vi "PV_DataLog.vi"(0 "Start 2":bool=TRUE, 2 "Start":bool=TRUE) -> ()   [LabVIEW 2016]
uses:
  <vilib>/Utility/file.llb/Write Delimited Spreadsheet (DBL).vi
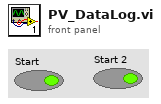
[diagram p1: front panel]
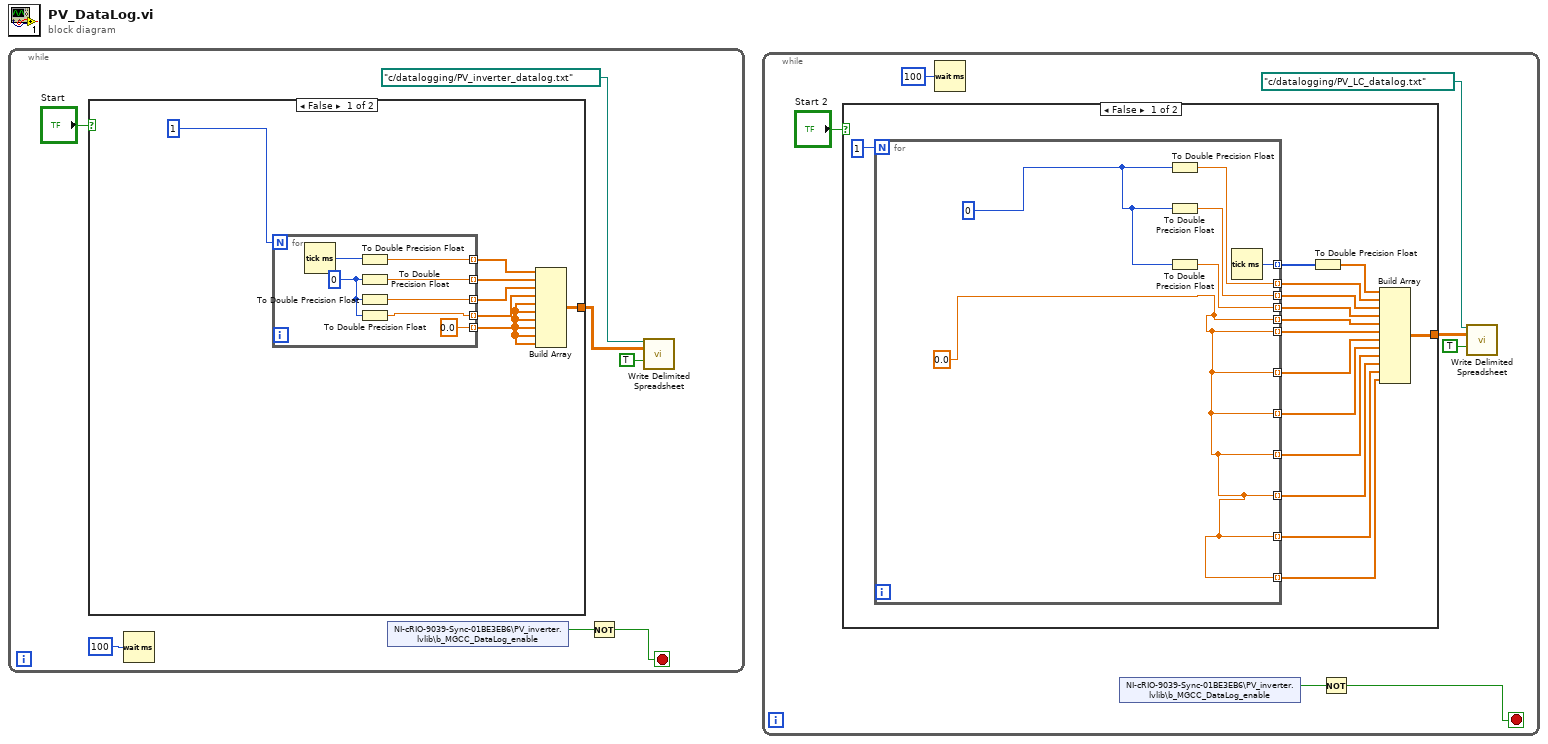
[diagram p0: block diagram]
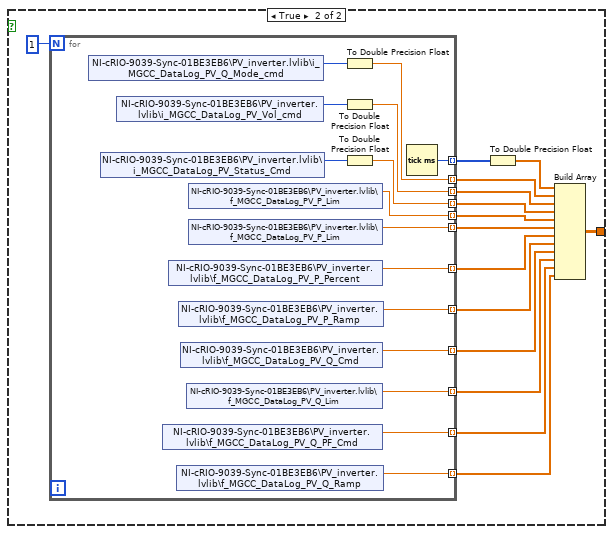
[diagram p2: hidden frame]
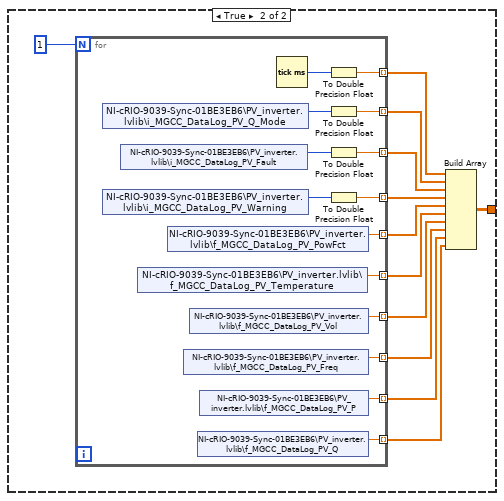
[diagram p3: hidden frame]
diagram:
  n1 = while {
    stop <- w1 stop-if-true
    n2 = case shown="False" "Start" {
      tunnel: [w9 w23] -> w4
      frame False {
        n3 = for {
          N: 1 -> [_]
          tunnel: [w21] -> w14 mode=indexing
          tunnel: [w19] -> w13 mode=indexing
          tunnel: [w18] -> w12 mode=indexing
          tunnel: [0.0] -> w11 mode=indexing
          tunnel: [w16] -> w10 mode=indexing
          w20 = 0
          n4 = Tick Count (ms)() -> (millisecond timer value=w15:u32)
          n5 = To Double Precision Float(number=w15) -> (double precision float=w16:dbl)
          n6 = To Double Precision Float(number=w20) -> (double precision float=w21:dbl)
          n7 = To Double Precision Float(number=w20) -> (double precision float=w19:dbl)
          n8 = To Double Precision Float(number=w20) -> (double precision float=w18:dbl)
        }
        n9 = Build Array(w10, w14, w13, w12, w11, w11, w11, w11, w11, w11) -> (w9:dbl[][])
      }
      frame True {
        n10 = for {
          N: 1 -> [_]
          tunnel: [w47] -> w33 mode=indexing
          tunnel: [w46] -> w32 mode=indexing
          tunnel: [w45] -> w31 mode=indexing
          tunnel: [w44] -> w30 mode=indexing
          tunnel: [w43] -> w29 mode=indexing
          tunnel: [w42] -> w28 mode=indexing
          tunnel: [w39] -> w27 mode=indexing
          tunnel: [w37] -> w26 mode=indexing
          tunnel: [w36] -> w25 mode=indexing
          tunnel: [w35] -> w24 mode=indexing
          n11 = shared-variable "NI-cRIO-9039-Sync-01BE3EB6\\PV_inverter.lvlib\\i_MGCC_DataLog_PV_Q_Mode"() -> (w41:i16)  [unwired: 1 in, 1 out]
          n12 = shared-variable "NI-cRIO-9039-Sync-01BE3EB6\\PV_inverter.lvlib\\i_MGCC_DataLog_PV_Warning"() -> (w38:i16)  [unwired: 1 in, 1 out]
          n13 = shared-variable "NI-cRIO-9039-Sync-01BE3EB6\\PV_inverter.lvlib\\i_MGCC_DataLog_PV_Fault"() -> (w40:i16)  [unwired: 1 in, 1 out]
          n14 = shared-variable "NI-cRIO-9039-Sync-01BE3EB6\\PV_inverter.lvlib\\f_MGCC_DataLog_PV_Temperature"() -> (w47:dbl)  [unwired: 1 in, 1 out]
          n15 = shared-variable "NI-cRIO-9039-Sync-01BE3EB6\\PV_inverter.lvlib\\f_MGCC_DataLog_PV_PowFct"() -> (w36:dbl)  [unwired: 1 in, 1 out]
          n16 = shared-variable "NI-cRIO-9039-Sync-01BE3EB6\\PV_inverter.lvlib\\f_MGCC_DataLog_PV_Freq"() -> (w45:dbl)  [unwired: 1 in, 1 out]
          n17 = shared-variable "NI-cRIO-9039-Sync-01BE3EB6\\PV_inverter.lvlib\\f_MGCC_DataLog_PV_Vol"() -> (w46:dbl)  [unwired: 1 in, 1 out]
          n18 = shared-variable "NI-cRIO-9039-Sync-01BE3EB6\\PV_inverter.lvlib\\f_MGCC_DataLog_PV_Q"() -> (w43:dbl)  [unwired: 1 in, 1 out]
          n19 = shared-variable "NI-cRIO-9039-Sync-01BE3EB6\\PV_inverter.lvlib\\f_MGCC_DataLog_PV_P"() -> (w44:dbl)  [unwired: 1 in, 1 out]
          n20 = Tick Count (ms)() -> (millisecond timer value=w34:u32)
          n21 = To Double Precision Float(number=w34) -> (double precision float=w35:dbl)
          n22 = To Double Precision Float(number=w41) -> (double precision float=w42:dbl)
          n23 = To Double Precision Float(number=w40) -> (double precision float=w39:dbl)
          n24 = To Double Precision Float(number=w38) -> (double precision float=w37:dbl)
        }
        n25 = Build Array(w24, w28, w27, w26, w25, w33, w32, w31, w30, w29) -> (w23:dbl[][])
      }
    }
    n26 = Wait (ms)(milliseconds to wait=u32 100) -> ()  [unwired: 1 out]
    n27 = shared-variable "NI-cRIO-9039-Sync-01BE3EB6\\PV_inverter.lvlib\\b_MGCC_DataLog_enable"() -> (w2:bool)  [unwired: 1 in, 1 out]
    n28 = Not(x=w2) -> (.not. x?=w1:bool)
    n29 = call-poly <vilib>:"Write Delimited Spreadsheet.vi"("file path (dialog if empty)"=path "c:/datalogging/PV_inverter_datalog.txt", "2D data"=w4, "append to file? (new file:F)"=TRUE) -> ()  [unwired: 11 in, 2 out]
  }
  n30 = while {
    stop <- w48 stop-if-true
    n31 = case shown="False" "Start 2" {
      tunnel: [w55 w83] -> w53
      frame False {
        n32 = for {
          N: 1 -> [_]
          tunnel: [w75] -> w57 mode=indexing
          tunnel: [w73] -> w59 mode=indexing
          tunnel: [w70] -> w68 mode=indexing
          tunnel: [w70] -> w67 mode=indexing
          tunnel: [w70] -> w66 mode=indexing
          tunnel: [w70] -> w65 mode=indexing
          tunnel: [w70] -> w64 mode=indexing
          tunnel: [w74] -> w63 mode=indexing
          tunnel: [w70] -> w62 mode=indexing
          tunnel: [w70] -> w61 mode=indexing
          tunnel: [w70] -> w60 mode=indexing
          tunnel: [w72] -> w58 mode=indexing
          w70 = 0.0
          w71 = 0
          n33 = To Double Precision Float(number=w71) -> (double precision float=w74:dbl)
          n34 = To Double Precision Float(number=w71) -> (double precision float=w73:dbl)
          n35 = To Double Precision Float(number=w71) -> (double precision float=w72:dbl)
          n36 = Tick Count (ms)() -> (millisecond timer value=w75:u32)
        }
        n37 = To Double Precision Float(number=w57) -> (double precision float=w56:dbl[])
        n38 = Build Array(w56, w63, w59, w58, w68, w67, w66, w65, w64, w62, w61, w60) -> (w55:dbl[][])
      }
      frame True {
        n39 = for {
          N: 1 -> [_]
          tunnel: [w105] -> w77 mode=indexing
          tunnel: [w92] -> w79 mode=indexing
          tunnel: [w104] -> w89 mode=indexing
          tunnel: [w103] -> w88 mode=indexing
          tunnel: [w102] -> w87 mode=indexing
          tunnel: [w101] -> w86 mode=indexing
          tunnel: [w100] -> w85 mode=indexing
          tunnel: [w93] -> w84 mode=indexing
          tunnel: [w99] -> w82 mode=indexing
          tunnel: [w98] -> w81 mode=indexing
          tunnel: [w97] -> w80 mode=indexing
          tunnel: [w91] -> w78 mode=indexing
          n40 = shared-variable "NI-cRIO-9039-Sync-01BE3EB6\\PV_inverter.lvlib\\i_MGCC_DataLog_PV_Q_Mode_cmd"() -> (w96:i16)  [unwired: 1 in, 1 out]
          n41 = shared-variable "NI-cRIO-9039-Sync-01BE3EB6\\PV_inverter.lvlib\\i_MGCC_DataLog_PV_Status_Cmd"() -> (w95:i16)  [unwired: 1 in, 1 out]
          n42 = shared-variable "NI-cRIO-9039-Sync-01BE3EB6\\PV_inverter.lvlib\\i_MGCC_DataLog_PV_Vol_cmd"() -> (w94:i16)  [unwired: 1 in, 1 out]
          n43 = shared-variable "NI-cRIO-9039-Sync-01BE3EB6\\PV_inverter.lvlib\\f_MGCC_DataLog_PV_Q_PF_Cmd"() -> (w98:dbl)  [unwired: 1 in, 1 out]
          n44 = shared-variable "NI-cRIO-9039-Sync-01BE3EB6\\PV_inverter.lvlib\\f_MGCC_DataLog_PV_P_Percent"() -> (w102:dbl)  [unwired: 1 in, 1 out]
          n45 = shared-variable "NI-cRIO-9039-Sync-01BE3EB6\\PV_inverter.lvlib\\f_MGCC_DataLog_PV_Q_Ramp"() -> (w97:dbl)  [unwired: 1 in, 1 out]
          n46 = shared-variable "NI-cRIO-9039-Sync-01BE3EB6\\PV_inverter.lvlib\\f_MGCC_DataLog_PV_P_Ramp"() -> (w101:dbl)  [unwired: 1 in, 1 out]
          n47 = shared-variable "NI-cRIO-9039-Sync-01BE3EB6\\PV_inverter.lvlib\\f_MGCC_DataLog_PV_Q_Cmd"() -> (w100:dbl)  [unwired: 1 in, 1 out]
          n48 = shared-variable "NI-cRIO-9039-Sync-01BE3EB6\\PV_inverter.lvlib\\f_MGCC_DataLog_PV_Q_Lim"() -> (w99:dbl)  [unwired: 1 in, 1 out]
          n49 = shared-variable "NI-cRIO-9039-Sync-01BE3EB6\\PV_inverter.lvlib\\f_MGCC_DataLog_PV_P_Lim"() -> (w104:dbl)  [unwired: 1 in, 1 out]
          n50 = shared-variable "NI-cRIO-9039-Sync-01BE3EB6\\PV_inverter.lvlib\\f_MGCC_DataLog_PV_P_Lim"() -> (w103:dbl)  [unwired: 1 in, 1 out]
          n51 = To Double Precision Float(number=w96) -> (double precision float=w93:dbl)
          n52 = To Double Precision Float(number=w94) -> (double precision float=w92:dbl)
          n53 = To Double Precision Float(number=w95) -> (double precision float=w91:dbl)
          n54 = Tick Count (ms)() -> (millisecond timer value=w105:u32)
        }
        n55 = To Double Precision Float(number=w77) -> (double precision float=w76:dbl[])
        n56 = Build Array(w76, w84, w79, w78, w89, w88, w87, w86, w85, w82, w81, w80) -> (w83:dbl[][])
      }
    }
    n57 = Wait (ms)(milliseconds to wait=u32 100) -> ()  [unwired: 1 out]
    n58 = shared-variable "NI-cRIO-9039-Sync-01BE3EB6\\PV_inverter.lvlib\\b_MGCC_DataLog_enable"() -> (w49:bool)  [unwired: 1 in, 1 out]
    n59 = Not(x=w49) -> (.not. x?=w48:bool)
    n60 = call-poly <vilib>:"Write Delimited Spreadsheet.vi"("file path (dialog if empty)"=path "c:/datalogging/PV_LC_datalog.txt", "2D data"=w53, "append to file? (new file:F)"=TRUE) -> ()  [unwired: 11 in, 2 out]
  }
